vi "rad_deg_conversion.vi"(1 "Rad":bool, 2 "InputString":string) -> (0 "result":string)   [LabVIEW 2015]
uses:
  <vilib>/regexp/Match Regular Expression.xnode
panel:
  # "If Rad = False, convert Degree to Rad\nif Rad = True, dont convert"
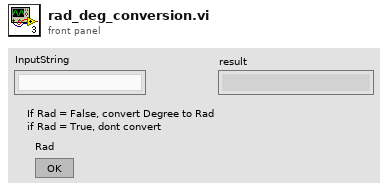
[diagram p1: front panel]
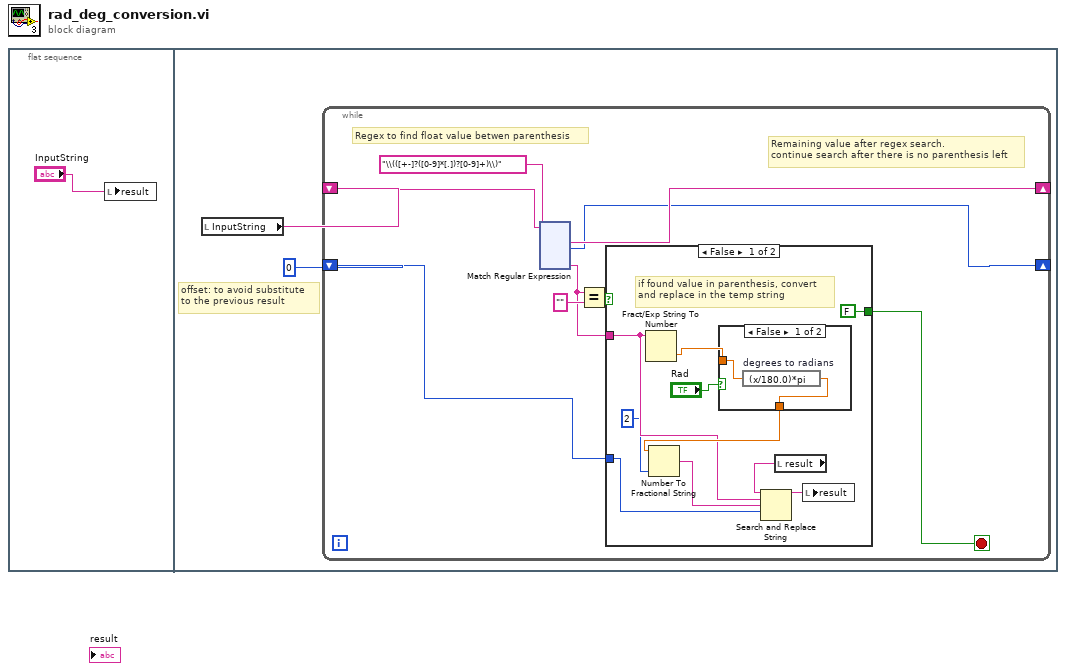
[diagram p0: block diagram]
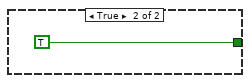
[diagram p3: hidden frame]
diagram:
  n1 = flat-sequence {
    frame #0 {
      n2 = local write "result"("InputString") -> ()
    }
    frame #1 {
      # "offset: to avoid substitute \nto the previous result"
      n3 = local read "InputString"() -> (w3:string)
      n4 = while {
        shift-right: [w10] -> _
        shift-left: w3 -> [w11]
        shift-right: [w4] -> _
        shift-left: 0 -> [w5]
        stop <- w7 stop-if-true
        # "Remaining value after regex search. \ncontinue search after there is no parenthesis left"
        # "Regex to find float value betwen parenthesis"
        n5 = xnode "Match Regular Expression"("input string"=w11, "regular expression"="\\(([+-]?([0-9]*[.])?[0-9]+)\\)") -> ("after match"=w10:string, "offset past match"=w4:i32, "submatch 1"=w6:string)  [unwired: 4 in, 3 out]
        n6 = Equal?(x=w6, y="") -> (x = y?=w8:bool)
        n7 = case shown="False" w8 {
          tunnel: [FALSE TRUE] -> w7
          tunnel: w6 -> [w17 _]
          tunnel: w5 -> [w14 _]
          frame False {
            # "if found value in parenthesis, convert\nand replace in the temp string"
            n8 = Fract/Exp String To Number(string=w17) -> (number=w22:dbl)  [unwired: 3 in, 1 out]
            n9 = case shown="False" "Rad" {
              tunnel: w22 -> [w24 w25]
              tunnel: [w23 w25] -> w21
              frame False {
                n10 = expression code="(x/180.0)*pi" "degrees to radians"(w24) -> (w23:dbl)
              }
              frame True {
              }
            }
            n11 = Number To Fractional String(number=w21, precision (6)=i16 2) -> (F-format string=w18:string)  [unwired: 2 in]
            n12 = local read "result"() -> (w20:string)
            n13 = Search and Replace String(input string=w20, search string=w17, replace string=w18, offset=w14) -> (result string=w19:string)  [unwired: 4 in, 3 out]
            n14 = local write "result"(w19) -> ()
          }
          frame True {
          }
        }
      }
    }
  }
